vi "PRACTICA 4 COMPUERTAS LOGICAS BASICAS.vi"() -> ()   [LabVIEW 2017]
panel:
  out "NOT":bool
  out "XOR":bool
  out "NOT AND":bool
  out "NOT OR":bool
  out "OR":bool
  out "AND":bool
  in  "BOTON B":bool
  in  "BOTON A":bool
  # "COMPUERTAS LOGICAS\nAND - OR - NOT OR - NOT AND - XOR - NOT"
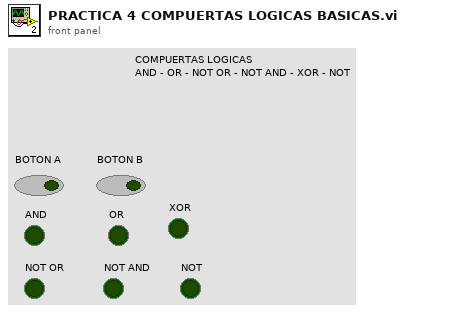
[diagram p1: front panel]
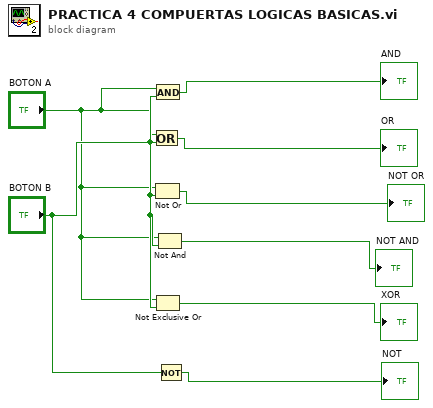
[diagram p0: block diagram]
diagram:
  n1 = Or(x="BOTON A", y="BOTON B") -> (x .or. y?=→"OR":bool)
  n2 = Not Or(1:"BOTON B", 2:"BOTON A") -> (0:→"NOT OR":bool)
  n3 = And(x="BOTON A", y="BOTON B") -> (x .and. y?=→"AND":bool)
  n4 = Not Exclusive Or(1:"BOTON B", 2:"BOTON A") -> (0:→"XOR":bool)
  n5 = Not And(1:"BOTON B", 2:"BOTON A") -> (0:→"NOT AND":bool)
  n6 = Not(x="BOTON B") -> (.not. x?=→"NOT":bool)
